vi "Proj (1).vi"() -> ()   [LabVIEW 2020]
panel:
  in  "stop":bool
  in  "Ring":u16(ring) items=["0", "1", "2", "3", "4", "5", "6", "7", "8", "9"]
  out "e":bool
  out "f":bool
  out "c":bool
  out "b":bool
  out "d":bool
  out "g":bool
  out "a":bool
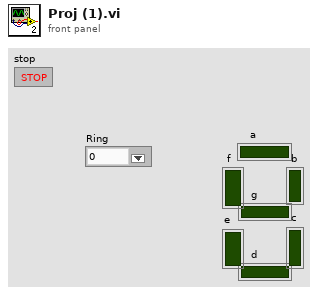
[diagram p1: front panel]
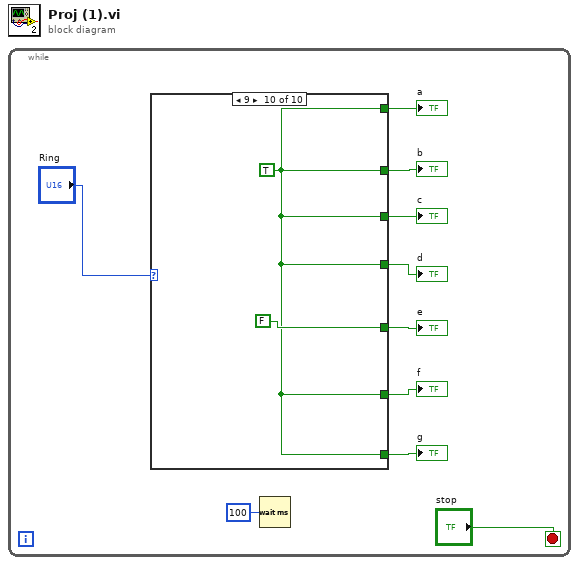
[diagram p0: block diagram]
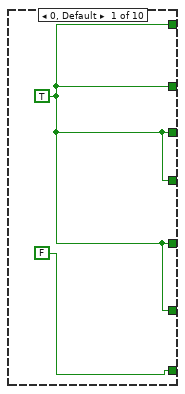
[diagram p2: hidden frame]
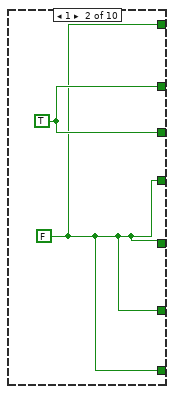
[diagram p3: hidden frame]
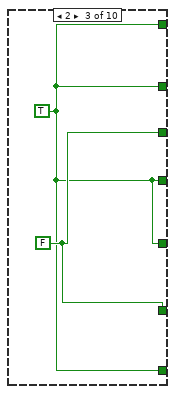
[diagram p4: hidden frame]
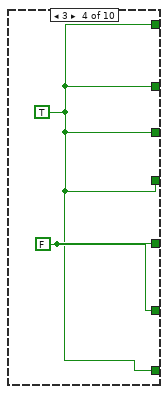
[diagram p5: hidden frame]
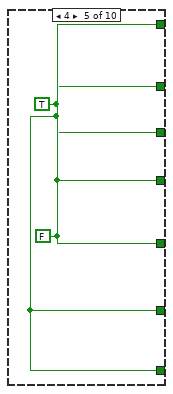
[diagram p6: hidden frame]
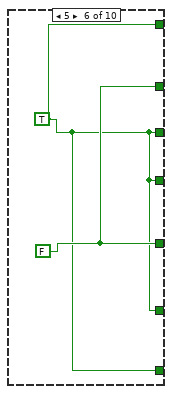
[diagram p7: hidden frame]
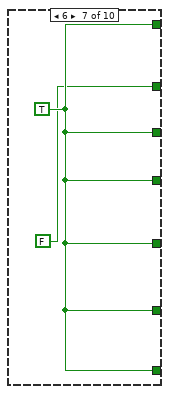
[diagram p8: hidden frame]
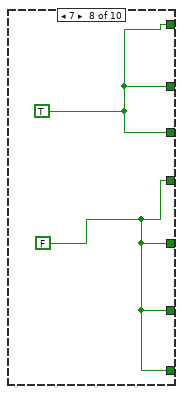
[diagram p9: hidden frame]
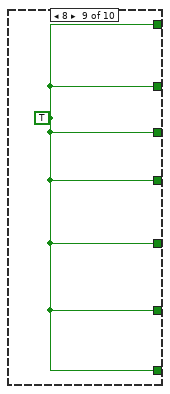
[diagram p10: hidden frame]
diagram:
  n1 = while {
    stop <- "stop" stop-if-true
    n2 = case shown="9" "Ring" {
      tunnel: [w11 w13 w15 w17 w20 w21 w24 w25 w27 w28] -> w9
      tunnel: [w11 w14 w15 w17 w19 w22 FALSE w25 w27 w28] -> w8
      tunnel: [w11 w14 w16 w17 w19 w21 w24 w25 w27 w28] -> w7
      tunnel: [w11 w13 w15 w17 w20 w21 w24 w26 w27 w28] -> w6
      tunnel: [w11 w13 w16 w18 w19 w21 w24 w26 w27 w28] -> w5
      tunnel: [FALSE w13 w15 w17 w19 w21 w24 w26 w27 w28] -> w4
      tunnel: [w11 w13 w15 w18 w20 w22 w24 w26 w27 FALSE] -> w3
      frame 0, Default {
        w11 = TRUE
      }
      frame 1 {
        w13 = FALSE
        w14 = TRUE
      }
      frame 2 {
        w16 = FALSE
        w15 = TRUE
      }
      frame 3 {
        w18 = FALSE
        w17 = TRUE
      }
      frame 4 {
        w20 = FALSE
        w19 = TRUE
      }
      frame 5 {
        w22 = FALSE
        w21 = TRUE
      }
      frame 6 {
        w24 = TRUE
      }
      frame 7 {
        w26 = FALSE
        w25 = TRUE
      }
      frame 8 {
        w27 = TRUE
      }
      frame 9 {
        w28 = TRUE
      }
    }
    "a" <- w9
    "g" <- w4
    "d" <- w6
    "b" <- w8
    "c" <- w7
    "f" <- w5
    "e" <- w3
    n3 = Wait (ms)(milliseconds to wait=u32 100) -> ()  [unwired: 1 out]
  }
